vi "SystemInfo.vi"(7 "LabVIEW Web Service Request":refnum<class "Web Request.lvclass">) -> ()   [LabVIEW 2013]
uses:
  <vilib>/wsapi/Web Request.lvclass
  <vilib>/NI/TagWebClient/API/JSON Formats/System Info Results.ctl
  <vilib>/Analysis/baseanly.llb/Mean (DBL).vi
  <vilib>/nisyscfg/Find Hardware.vi
  <vilib>/Analysis/NI_AALBase.lvlib
  <vilib>/NI/TagWebClient/API/tagweb client API.lvlib
  <vilib>/nisyscfg/nisyscfg.lvlib
panel:
  # "Use the Web Service Request input terminal to call the VIs on the Web Services palette. Do not remove it from the connector pane unless you don't need access to the palette."
  # "Each additional control wired to the connector pane will be available as an input in the URL. To include an indicator in terminal-mode output (the default setting), it must also be wired to the connector pane."
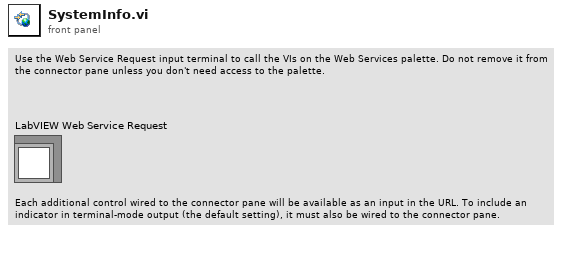
[diagram p1: front panel]
types:
  T1 = typedef "tagweb client API.lvlib/System Info Results.ctl" = cluster{"CPU":dbl, "FreeMemory":dbl, "TotalMemory":dbl, "FreeMemoryPercent":dbl}
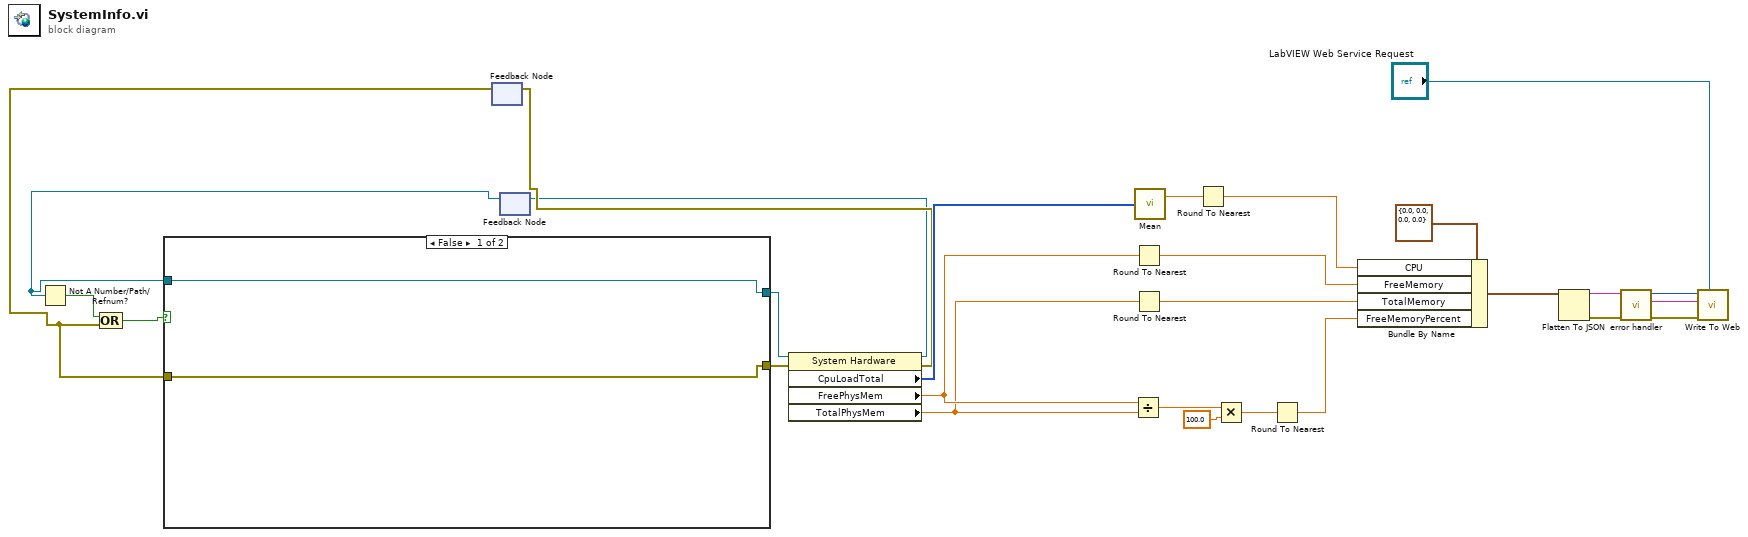
[diagram p0: block diagram]
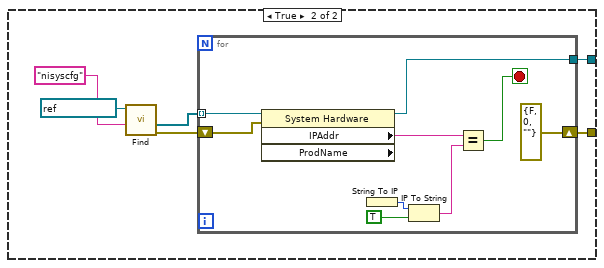
[diagram p2: hidden frame]
diagram:
  n1 = feedback #1() -> (w2:errorcluster)  [unwired: 1 in]
  n2 = feedback #2() -> (w1:refnum<k20>)  [unwired: 1 in]
  n3 = Not A Number/Path/Refnum?(number/path/refnum=w1) -> (NaN/Path/Refnum?=w4:bool)
  n4 = Compound Arithmetic op=OR(w4, w2) -> (w3:bool)
  n5 = case shown="False" w3 {
    tunnel: [w28 w33] -> w8
    tunnel: [w29 w32] -> w7
    tunnel: w2 -> [w29 _]
    tunnel: w1 -> [w28 _]
    frame False {
    }
    frame True {
      n6 = call-poly <vilib>:"Find.vi"("experts"="nisyscfg", "session in"=refnum<k21> "localhost") -> ("error out"=w31:errorcluster, "resources out"=w34:refnum<k20>[])  [unwired: 6 in, 2 out]
      n7 = for {
        tunnel: w34 -> [w44] mode=indexing
        tunnel: [w39] -> w33
        shift-right: [errorcluster {"status"=FALSE, "code"=0, "source"=""} ("error out")] -> w32
        shift-left: w31 -> [w37]
        stop <- w38 stop-if-true
        n8 = property class="System Hardware" props=["IPAddr", "ProdName"](reference=w44, error in=w37) -> (reference out=w39:refnum<k20>, "IPAddr"=w41:string)  [unwired: 2 out]
        n9 = String To IP() -> (0:w42:u32)  [unwired: 1 in]
        n10 = IP To String(1:TRUE ("dot notation? (F)"), 2:w42) -> (0:w40:string)
        n11 = Equal?(x=w41, y=w40) -> (x = y?=w38:bool)
      }
    }
  }
  n12 = property class="System Hardware"(reference=w8, error in=w7) -> (reference out=w6:refnum<k20>, error out=w9:errorcluster, "CpuLoadTotal"=w16:u32[], "FreePhysMem"=w14:dbl, "TotalPhysMem"=w13:dbl)
  n13 = feedback-in #1(w9) -> ()
  n14 = feedback-in #2(w6) -> ()
  n15 = Divide(x=w14, y=w13) -> (x/y=w12:dbl)
  n16 = Round To Nearest(number=w14) -> (nearest integer value=w20:dbl)
  n17 = Round To Nearest(number=w13) -> (nearest integer value=w19:dbl)
  n18 = call-poly <vilib>:"Mean.vi"("X"=w16) -> ("mean"=w15:dbl)  [unwired: 1 out]
  n19 = Round To Nearest(number=w15) -> (nearest integer value=w17:dbl)
  n20 = Multiply(x=w12, y=100.0) -> (x*y=w10:dbl)
  n21 = Round To Nearest(number=w10) -> (nearest integer value=w18:dbl)
  n22 = Bundle By Name(cluster=T1 {"CPU"=0.0, "FreeMemory"=0.0, "TotalMemory"=0.0, "FreeMemoryPercent"=0.0} ("System Info"), "CPU"=w17, "FreeMemory"=w20, "TotalMemory"=w19, "FreeMemoryPercent"=w18) -> (w5:T1)
  n23 = Flatten To JSON(anything=w5) -> (JSON string=w27:string, 11:w26:errorcluster)  [unwired: 2 in]
  n24 = call "error handler.vi"("error in (no error)"=w26, "Success Message"=w27) -> ("error out"=w25:errorcluster, "Response String"=w22:string, "Response Code"=w23:i32)  [unwired: 7 in]
  n25 = call <vilib>:"Write To Web.vi"("Web Request in"="LabVIEW Web Service Request", "error in (no error)"=w25, "Response String"=w22, "Response Code"=w23) -> ()  [unwired: 7 in, 1 out]
